vi "Actor Core.vi"(8 "error in":errorcluster, 11 "Stage in":refnum<class "Stage.lvclass">) -> (0 "error out":errorcluster, 3 "Actor out":refnum<class "Actor.lvclass">)   [LabVIEW 2020, in "Stage.lvlib" / "Stage.lvclass"]
doc: "(<B>Filename</B>: Actor Framework.lvlib:Actor.lvclass:Actor Core.vi)\n\nReceives messages to the actor, reacts to them, and initiates any error handling that may shut the actor down.\n\nDescendant classes may override this VI to append parallel tasks for the actor to complete while it handles messages. Overrides use the Call Parent Class Method node."
uses:
  Stage.lvclass
  C:/Program Files/National Instruments/LabVIEW 2020/vi.lib/ActorFramework/Actor/Actor.lvclass
  <vilib>/ActorFramework/Actor/Actor.lvclass
  Controller/Stage Controller/Stage Controller.lvclass
  Controller/Stage Controller StepMotor/Stage Controller StepMotor.lvclass
  Stage.lvclass/Stage.ctl
  Device/Device/Device.lvclass
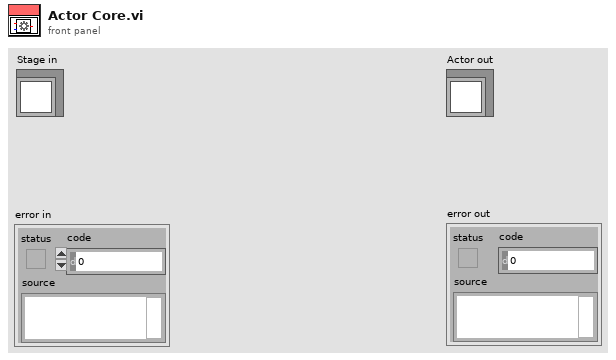
[diagram p1: front panel]
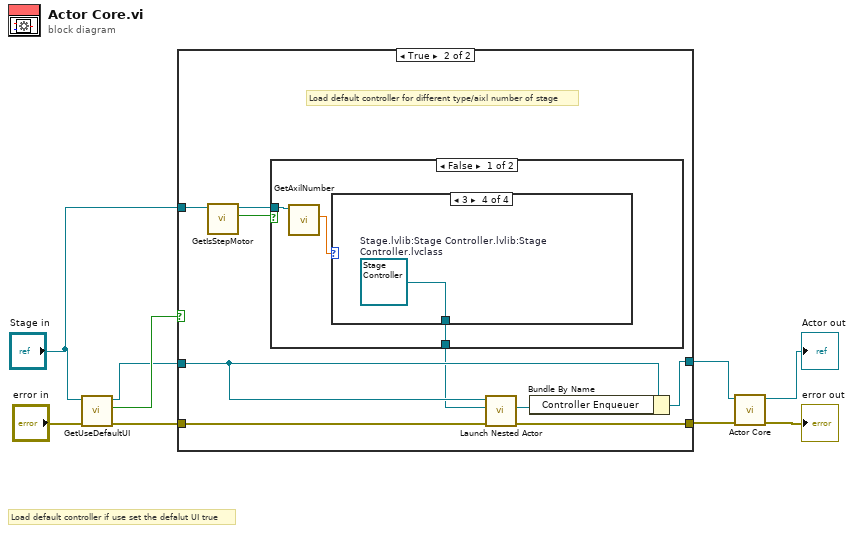
[diagram p0: block diagram]
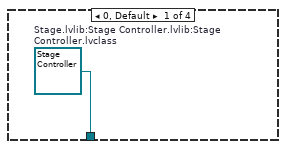
[diagram p3: hidden frame]
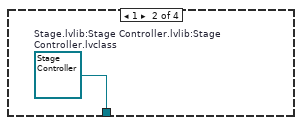
[diagram p4: hidden frame]
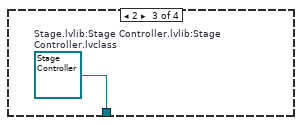
[diagram p5: hidden frame]
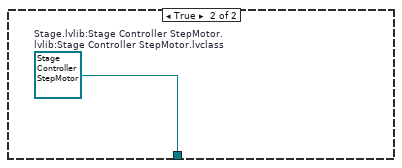
[diagram p6: hidden frame]
diagram:
  # "Load default controller if use set the defalut UI true"
  n1 = call-dynamic "GetUseDefaultUI.vi"("error in (no error)"="error in", "Device in"="Stage in") -> ("error out"=w5:errorcluster, "User Default UI?"=w6:bool, "Device out"=w4:refnum<class "Stage.lvclass">)  [unwired: 7 in]
  n2 = case shown="True" w6 {
    tunnel: "Stage in" -> [_ w20]
    tunnel: w5 -> [w10 w16]
    tunnel: w4 -> [w11 w13]
    tunnel: [w11 w14] -> w3
    tunnel: [w10 w15] -> w2
    frame False {
    }
    frame True {
      # "Load default controller for different type/aixl number of stage"
      n3 = call-dynamic "GetIsStepMotor.vi"("Stage in"=w20) -> ("IsStepMotor?"=w18:bool, "Stage out"=w19:refnum<class "Stage.lvclass">)  [unwired: 8 in, 1 out]
      n4 = case shown="False" w18 {
        tunnel: [w23 w28] -> w12
        tunnel: w19 -> [w22 _]
        frame False {
          n5 = call-dynamic "GetAxilNumber.vi"("Stage in"=w22) -> ("Axil Number"=w21:dbl)  [unwired: 8 in, 2 out]
          n6 = case shown="3" w21 {
            tunnel: [w24 w25 w26 w27] -> w23
            frame 0, Default {
              w24 = refnum<class "Stage Controller.lvclass"> refnum  # Stage.lvlib:Stage Controller.lvlib:Stage Controller.lvclass
            }
            frame 1 {
              w25 = refnum<class "Stage Controller.lvclass"> refnum  # Stage.lvlib:Stage Controller.lvlib:Stage Controller.lvclass
            }
            frame 2 {
              w26 = refnum<class "Stage Controller.lvclass"> refnum  # Stage.lvlib:Stage Controller.lvlib:Stage Controller.lvclass
            }
            frame 3 {
              w27 = refnum<class "Stage Controller.lvclass"> refnum  # Stage.lvlib:Stage Controller.lvlib:Stage Controller.lvclass
            }
          }
        }
        frame True {
          w28 = refnum<class "Stage Controller StepMotor.lvclass"> refnum  # Stage.lvlib:Stage Controller StepMotor.lvlib:Stage Controller StepMotor.lvclass
        }
      }
      n7 = call <vilib>:"Launch Nested Actor.vi"("error in (no error)"=w16, "Nested Actor"=w12, "Caller Actor in"=w13) -> ("error out"=w15:errorcluster, "Nested Actor's Enqueuer"=w17:refnum<class "Message Enqueuer.lvclass">)  [unwired: 6 in, 1 out]
      n8 = Bundle By Name(cluster=w13, "Controller Enqueuer"=w17) -> (w14:refnum<class "Stage.lvclass">)
    }
  }
  n9 = call-parent "Actor Core.vi"("error in"=w2, "Actor in"=w3) -> ("error out"=→"error out":errorcluster, "Actor out"=→"Actor out":refnum<class "Actor.lvclass">)  [unwired: 8 in]
